vi "SCC File History.vi"(6 "versions":string[](array[string]), 7 "advanced options":variant, 8 "error in (no error)":errorcluster, 10 "files":path[](array[path]), 11 "source control reference in":T1) -> (0 "error out":errorcluster, 2 "status message":string, 3 "source control reference out":T1, 5 "file changed?":bool)   [LabVIEW 2017, in "NI_SCC.lvlib"]
doc: "Returns the source control history for specified files. The source control history provides information about previous versions of the files."
uses:
  <vilib>/SourceControl/sccapi/NI_SCC.lvlib
  <vilib>/SourceControl/sccapi/SCCAPI Refnum.ctl
  <vilib>/SourceControl/sccapi/SCCAPI SCC Operations.ctl
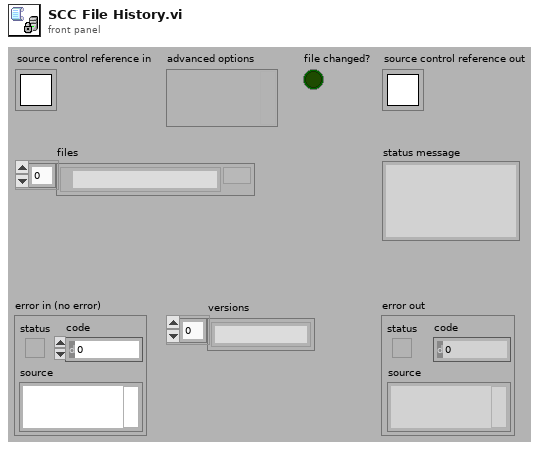
[diagram p1: front panel]
types:
  T1 = typedef "NI_SCC.lvlib/SCCAPI Refnum.ctl" = refnum<k1>
  T2 = typedef "NI_SCC.lvlib/SCCAPI SCC Operations.ctl" = enum16{"Add", "Check In", "Check Out", "Close Project", "Compare Files", "Compare VIs", "Configure Project", "File History", "File Properties", "File Status", "Find All Providers", "Get Advanced Command Options", "Get File Copy", "Get Latest Version", "Get Project Name", "Get StaticVI Path", "Initialize", "Not A Source Control Reference", "Open Project", "Provider Supports Functionality", "Remove", "Run Provider", "Undo Check Out", "Uninitialize", "Is File In Local Path"}
  T3 = typedef "SCCAPI Refnum.ctl" = refnum<k1>
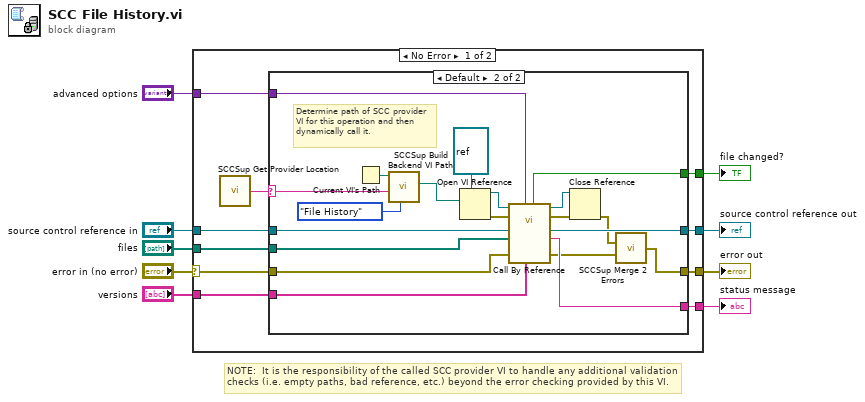
[diagram p0: block diagram]
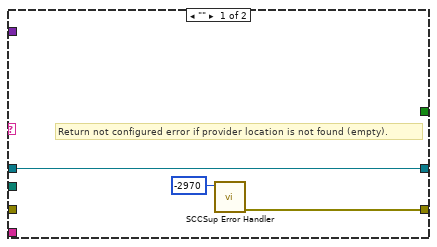
[diagram p2: hidden frame]
diagram:
  # "NOTE:  It is the responsibility of the called SCC provider VI to handle any additional validation checks (i.e. empty paths, bad reference, etc.) beyond the error checking provided by this VI."
  n1 = case shown="No Error" "error in (no error)" {
    selector: "error in (no error)" -> [w11 w44]
    tunnel: [w19 w44] -> w8
    tunnel: "source control reference in" -> [w18 w43]
    tunnel: [w17 _] -> w6
    tunnel: [w16 w43] -> w5
    tunnel: "files" -> [w15 _]
    tunnel: "versions" -> [w14 _]
    tunnel: [w12 _] -> w2
    tunnel: "advanced options" -> [w10 _]
    frame No Error {
      n2 = call <vilib>:"SCCSup Get Provider Location.vi"() -> ("provider location"=w13:string)  [unwired: 6 in]
      n3 = case shown="Default" w13 {
        selector: w13 -> [_ w26]
        tunnel: [w20 w42] -> w19
        tunnel: w18 -> [w22 w34]
        tunnel: [_ w41] -> w17
        tunnel: [w22 w35] -> w16
        tunnel: w15 -> [_ w33]
        tunnel: w14 -> [_ w32]
        tunnel: [_ w25] -> w12
        tunnel: w11 -> [_ w24]
        tunnel: w10 -> [_ w23]
        frame "" {
          # "Return not configured error if provider location is not found (empty)."
          n4 = call <vilib>:"SCCSup Error Handler.vi"("scc error code"=-2970 ("code")) -> ("error out"=w20:errorcluster)  [unwired: 10 in]
        }
        frame Default {
          # "Determine path of SCC provider VI for this operation and then dynamically call it."
          n5 = Current VI's Path() -> (path=w29:path)
          n6 = call <vilib>:"SCCSup Build Backend VI Path.vi"("scc operation"=SCCAPI_SCC_Operations."File History", "provider location"=w26, "caller path"=w29) -> ("scc backend VI path"=w28:path)  [unwired: 8 in]
          n7 = Open VI Reference(type specifier VI Refnum (for type only)=refnum<vi> refnum, vi path=w28) -> (vi reference=w39:refnum<vi>, error out=w38:errorcluster)  [unwired: 4 in]
          n8 = call-by-ref "?"(reference=w39, error in=w38, "versions"=w32, "advanced options"=w23, "error in (no error)"=w24, "files"=w33, "source control reference in"=w34) -> (reference out=w37:refnum<vi>, error out=w36:errorcluster, 0:"error out"=w30:errorcluster, "status message"=w41:string, "source control reference out"=w35:T3, "file changed?"=w25:bool)  [unwired: 3 in]
          n9 = Close Reference(reference=w37, error in (no error)=w36) -> (error out=w31:errorcluster)
          n10 = call <vilib>:"SCCSup Merge 2 Errors.vi"("Error IO 1"=w31, "Error IO 2"=w30) -> ("Error IO out"=w42:errorcluster)  [unwired: 13 in]
        }
      }
    }
    frame Error {
    }
  }
  "error out" <- w8
  "status message" <- w6
  "source control reference out" <- w5
  "file changed?" <- w2
